vi "Timon_Kerto.vi"(8 "error in (no error)":errorcluster, 10 "Number 2":dbl, 11 "Number 1":dbl) -> (0 "error out":errorcluster, 3 "Sum":dbl)   [LabVIEW 2019]
doc: "Version 1.0.0.0 8.10.2020\nKONE Corporation\nAll Rights Reserved\n\n<description of the VI functionality and purpose>\n\nVersion History\n---------------------\n1.0.0.0 - Original VI\n1.0.x.x - The changes made"
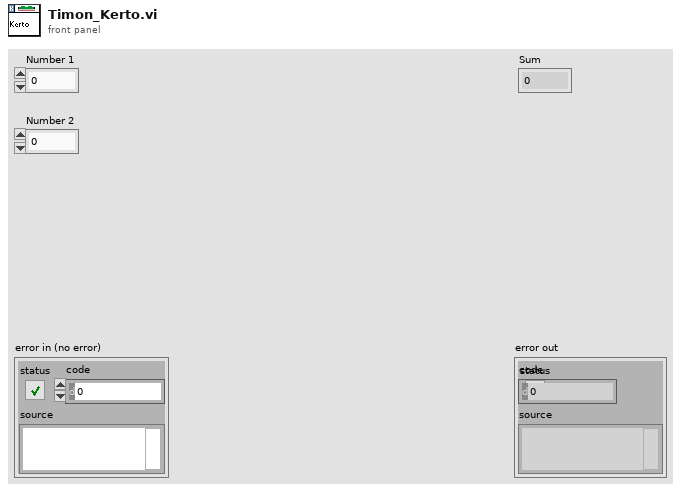
[diagram p1: front panel]
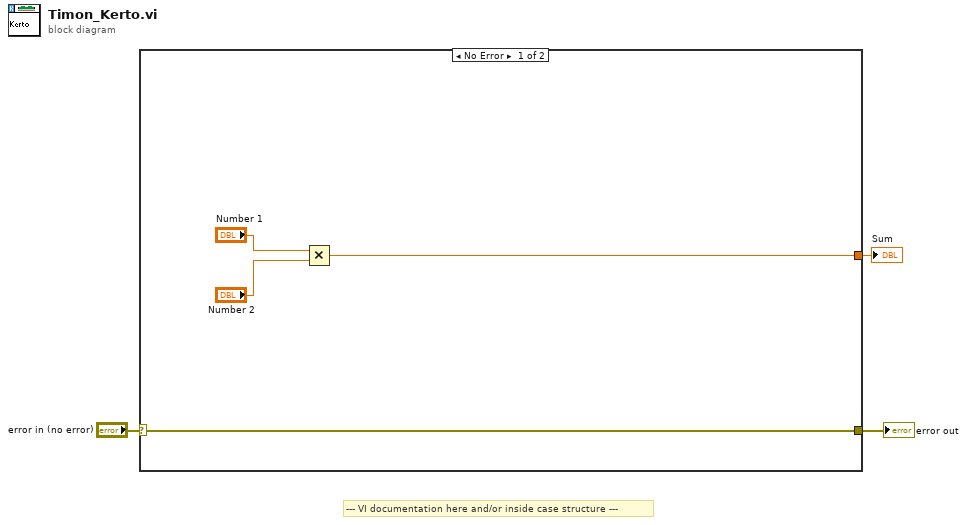
[diagram p0: block diagram]
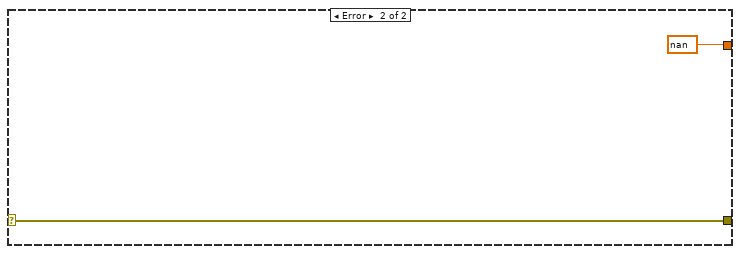
[diagram p2: hidden frame]
diagram:
  # "--- VI documentation here and/or inside case structure ---"
  n1 = case shown="No Error" "error in (no error)" {
    selector: "error in (no error)" -> [w5 w9]
    tunnel: [w5 w9] -> w2
    tunnel: [w4 nan] -> w1
    frame No Error {
      n2 = Multiply(x="Number 1", y="Number 2") -> (x*y=w4:dbl)
    }
    frame Error {
    }
  }
  "error out" <- w2
  "Sum" <- w1
